vi "CRYPIC Update View.vi"(9 "sTitle":string, 10 "pVIRef":refnum<vi>) -> ()   [LabVIEW 2013]
uses:
  DataView/VIEW/CRYNew View Global.vi
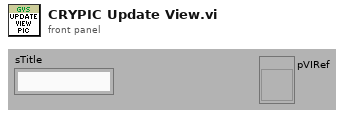
[diagram p1: front panel]
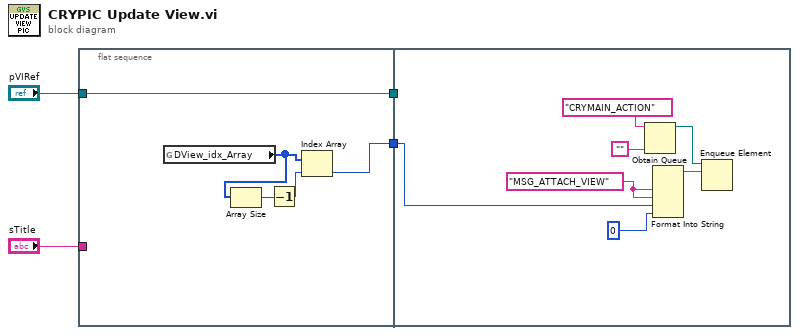
[diagram p0: block diagram]
diagram:
  n1 = flat-sequence {
    tunnel: "pVIRef" -> [w9]
    tunnel: [w9] -> w4
    tunnel: [w8] -> w3
    tunnel: "sTitle" -> [_]
    tunnel: w3 -> [w10]
    tunnel: w4 -> [_]
    frame #0 {
      n2 = global read "CRYNew View Global.vi" "DView_idx_Array"() -> (w7:i32[])
      n3 = Array Size(array=w7) -> (size(s)=w6:i32)
      n4 = Decrement(x=w6) -> (x-1=w5:i32)
      n5 = Index Array(array=w7, index=w5) -> (element=w8:i32)
    }
    frame #1 {
      w12 = "MSG_ATTACH_VIEW" ("input 1")
      n6 = Obtain Queue(name (unnamed)="CRYMAIN_ACTION" ("YAxisTitle"), element data type="" ("Action Type")) -> (queue out=w13:refnum<queue>)  [unwired: 3 in, 2 out]
      n7 = Format Into String(w12, w12, w10, 0 ("input 3")) -> (resulting string=w14:string)  [unwired: 3 in, 1 out]
      n8 = Enqueue Element(queue=w13, element=w14) -> ()  [unwired: 1 in, 4 out]
    }
  }
